vi "Update_Simon_Scores.vi"(9 "Score":i32, 10 "Position":i32, 11 "LoopLength":i32) -> (1 "New Score":i32, 2 "Next Pos":i32, 3 "Case Selector":i32)   [LabVIEW 2025]
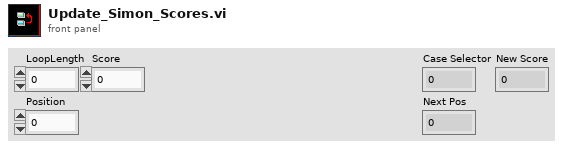
[diagram p1: front panel]
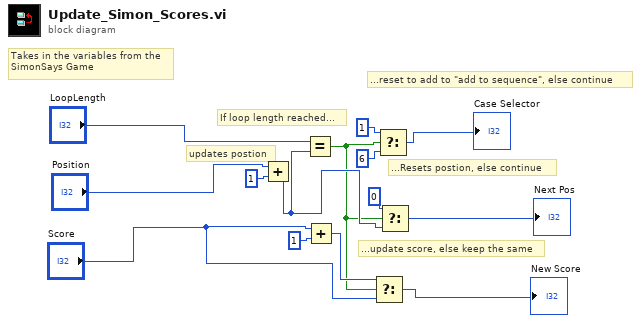
[diagram p0: block diagram]
diagram:
  # "If loop length reached..."
  # "...update score, else keep the same"
  # "...reset to add to \"add to sequence\", else continue"
  # "...Resets postion, else continue"
  # "updates postion"
  # "Takes in the variables from the\nSimonSays Game"
  n1 = Add(x="Position", y=1) -> (x+y=w10:i32)
  n2 = Equal?(x="LoopLength", y=w10) -> (x = y?=w7:bool)
  n3 = Add(x="Score", y=1) -> (x+y=w8:i32)
  n4 = Select(t=w8, s=w7, f="Score") -> (s? t:f=→"New Score":i32)
  n5 = Select(t=1 ("f"), s=w7, f=6) -> (s? t:f=→"Case Selector":i32)
  n6 = Select(t=0 ("f"), s=w7, f=w10) -> (s? t:f=→"Next Pos":i32)
